vi "Testing Keithley.vi"() -> ()   [LabVIEW 2017]
panel:
  in  "String":string
  in  "function (Vdc:1)":u16(ring)=1 items=["ac voltage", "dc voltage", "2-wire resistance", "4-wire resistance", "ac current", "dc current", "frequency", "temperature"]
  out "Reading Result":string
  in  "error in":T1
  out "error out":T1
  in  "GPIB Address":string
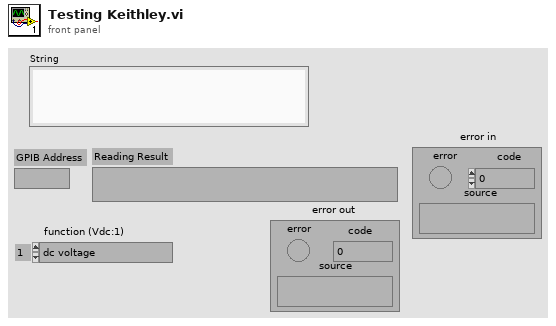
[diagram p1: front panel]
types:
  T1 = cluster{"error":bool, "code":i32, "source":string}
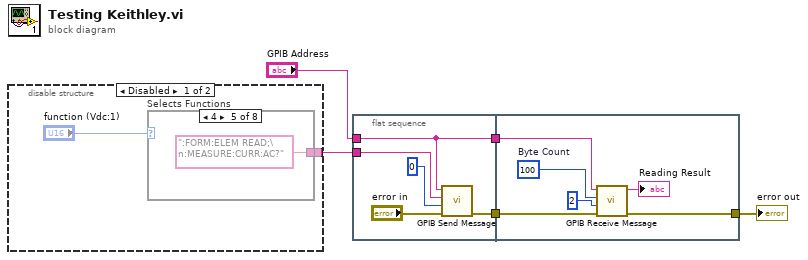
[diagram p0: block diagram]
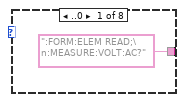
[diagram p2: hidden frame]
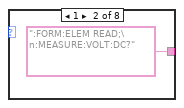
[diagram p3: hidden frame]
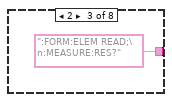
[diagram p4: hidden frame]
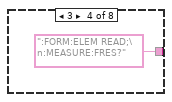
[diagram p5: hidden frame]
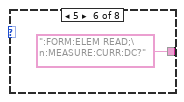
[diagram p6: hidden frame]
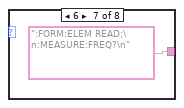
[diagram p7: hidden frame]
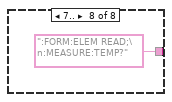
[diagram p8: hidden frame]
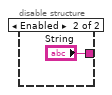
[diagram p9: hidden frame]
diagram:
  n1 = disable-structure shown="Disabled" {
    disable-tunnel: [w6 "String"] -> w4
    frame Disabled {
      n2 = case "Selects Functions" shown="4" "function (Vdc:1)" {
        tunnel: [":FORM:ELEM READ;\n:MEASURE:VOLT:AC?" ":FORM:ELEM READ;\n:MEASURE:VOLT:DC?" ":FORM:ELEM READ;\n:MEASURE:RES?" ":FORM:ELEM READ;\n:MEASURE:FRES?" ":FORM:ELEM READ;\n:MEASURE:CURR:AC?" ":FORM:ELEM READ;\n:MEASURE:CURR:DC?" ":FORM:ELEM READ;\n:MEASURE:FREQ?\n" ":FORM:ELEM READ;\n:MEASURE:TEMP?"] -> w6
        frame ..0 {
        }
        frame 1 {
        }
        frame 2 {
        }
        frame 3 {
        }
        frame 4 {
        }
        frame 5 {
        }
        frame 6 {
        }
        frame 7.. {
        }
      }
    }
    frame Enabled {
    }
  }
  n3 = flat-sequence {
    tunnel: "GPIB Address" -> [w21]
    tunnel: [w21] -> w3
    tunnel: w4 -> [w18]
    tunnel: [w17] -> w2
    tunnel: w3 -> [w27]
    tunnel: w2 -> [w23]
    tunnel: [w22] -> w1
    frame #0 {
      n4 = call "GPIB Send Message.vi"("address string"=w21, "write buffer"=w18, "write mode (set END:0)"=0, "error in"="error in") -> ("error out"=w17:T1)  [unwired: 3 in, 2 out]
    }
    frame #1 {
      w26 = 100  # Byte Count
      n5 = call "GPIB Receive Message.vi"("address string"=w27, "byte count"=w26, "read mode"=2, "error in"=w23) -> ("read buffer"=→"Reading Result":string, "error out"=w22:T1)  [unwired: 3 in, 1 out]
    }
  }
  "error out" <- w1
